vi "ExecuteMenuCommand.vi"(0 "reference in":refnum<class "VINode.lvclass">, 1 "Command":string, 5 "error in (no error)":errorcluster) -> (14 "reference out":refnum<class "VINode.lvclass">, 15 "EditorAction":T3, 16 "FlattenCommandSettings":T1, 19 "error out":errorcluster)   [LabVIEW 2014, in "VINode.lvclass"]
uses:
  <resource>/Framework/Providers/Open_GDS/UML/VINode_class/VINode.lvclass
  <resource>/Framework/Providers/Open_GDS/UML/UMLEditor/UMLEditor EditorActionType.ctl
  <resource>/Framework/Providers/Open_GDS/UML/UMLEditor/UMLEditor FlattenCommandType.ctl
  <resource>/Framework/Providers/Open_GDS/UML/UMLEditor/UMLEditor ExecuteCommandType.ctl
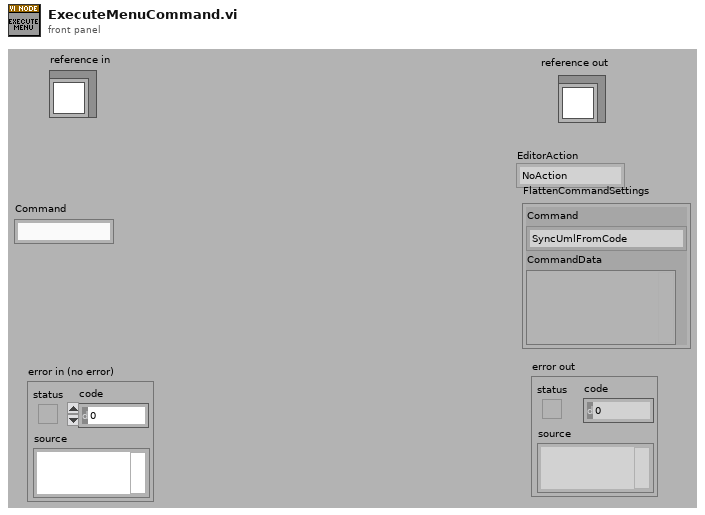
[diagram p1: front panel]
types:
  T1 = typedef "UMLEditor FlattenCommandType.ctl" = cluster{"Command":T2, "CommandData":variant}
  T2 = typedef "UMLEditor ExecuteCommandType.ctl" = enum16{"SyncUmlFromCode", "SyncCodeFromUML", "OpenClass", "OpenFile", "CreateClass", "CreateVI", "OpenClassAttribute", "LocateInProject"}
  T3 = typedef "UMLEditor EditorActionType.ctl" = enum16{"NoAction", "Repaint", "ExecuteCommand"}
  T4 = typedef "VINode.lvclass/ObjectAttributes.ctl" = cluster{"midHeight":dbl, "botHeight":dbl, "Name":refnum<class "MultiLineString.lvclass">, "DEFAULT_COMPARTMENT_HEIGHT":i32, "DEFAULT_WIDTH":i32, "DEFAULT_HEIGHT":i32, "ClassPath":path, "Icon":u8[][], "Description":refnum<class "MultiLineString.lvclass">, "ShowDescription":bool}
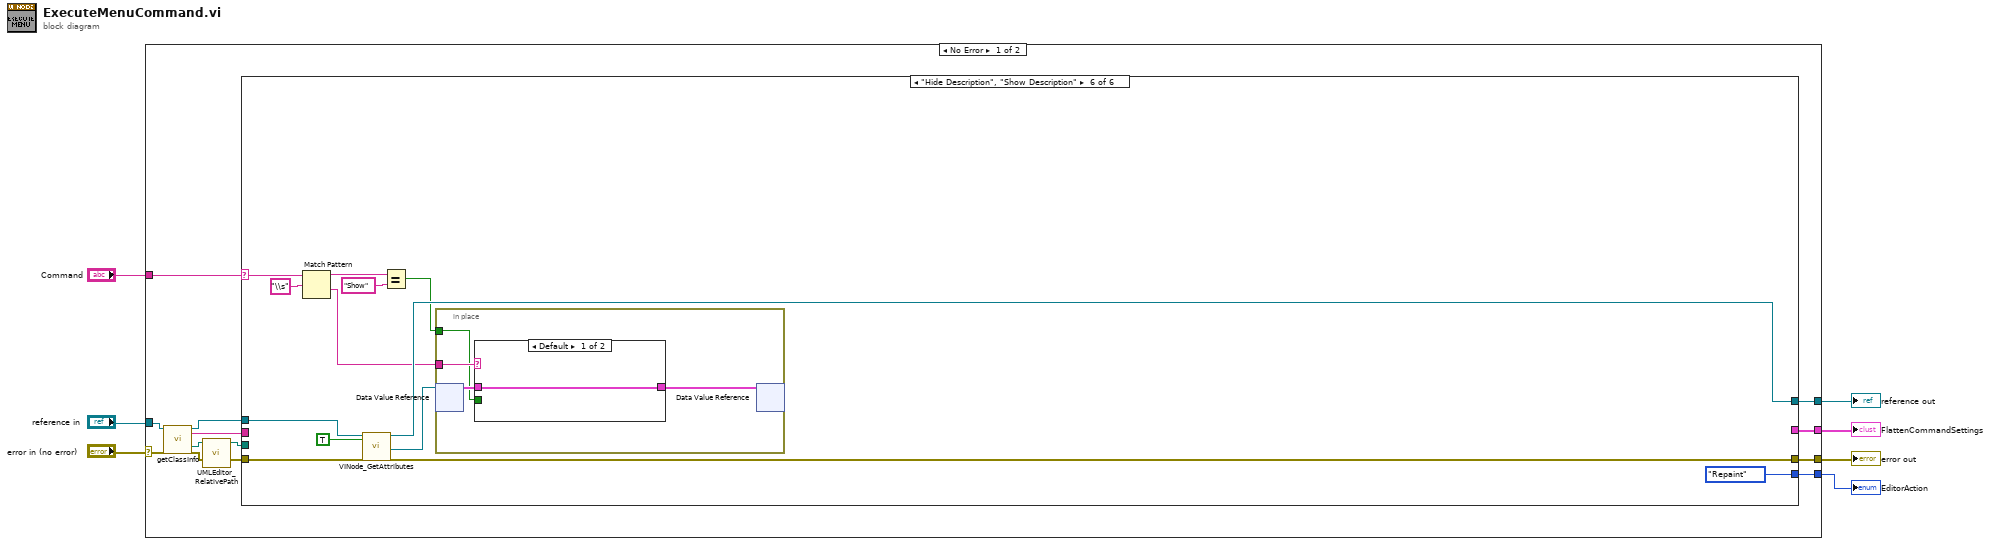
[diagram p0: block diagram]
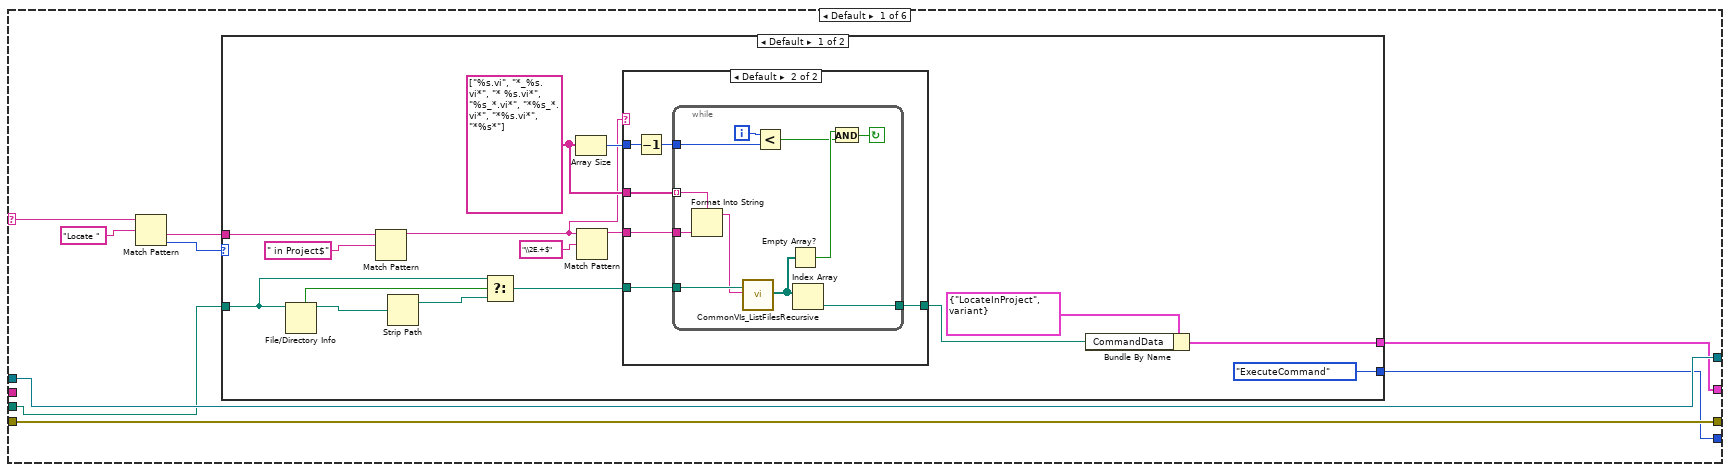
[diagram p2: hidden frame]
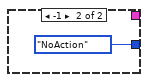
[diagram p4: hidden frame]
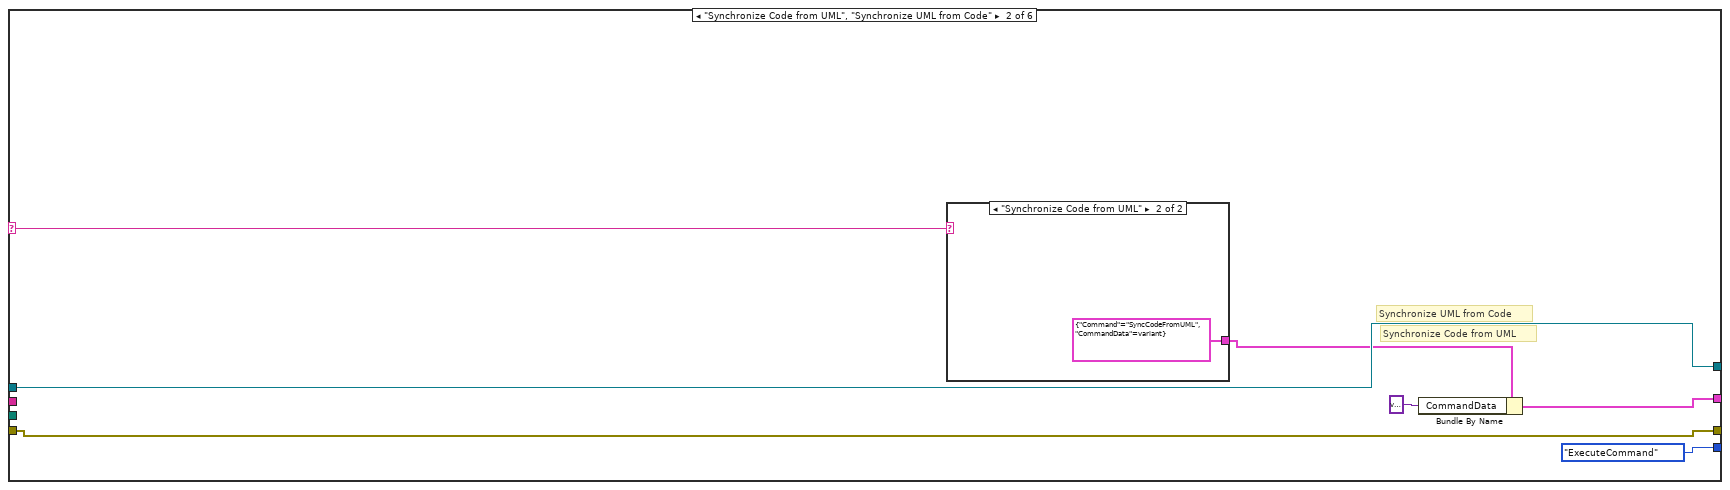
[diagram p5: hidden frame]
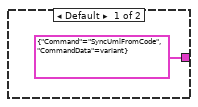
[diagram p6: hidden frame]
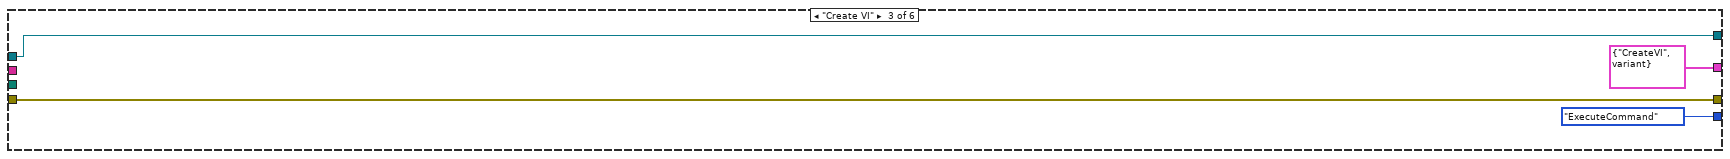
[diagram p7: hidden frame]
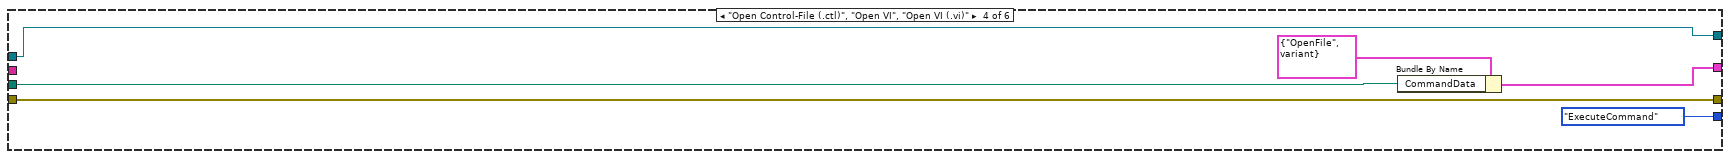
[diagram p8: hidden frame]
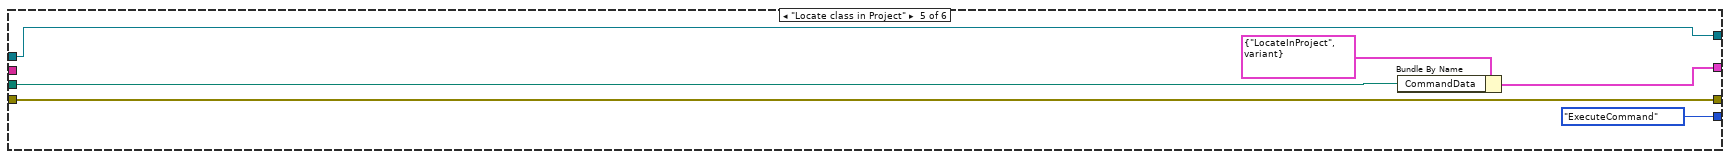
[diagram p9: hidden frame]
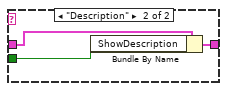
[diagram p10: hidden frame]
diagram:
  n1 = case shown="No Error" "error in (no error)" {
    selector: "error in (no error)" -> [w12 w109]
    tunnel: "reference in" -> [w14 w110]
    tunnel: [w17 w109] -> w5
    tunnel: [w18 w110] -> w4
    tunnel: "Command" -> [w19 _]
    tunnel: [w16 _] -> w2
    tunnel: [w15 _] -> w1
    frame No Error {
      n2 = call-dynamic "getClassInfo.vi"("reference in"=w14, "error in (no error)"=w12) -> ("reference out"=w13:refnum<class "VINode.lvclass">, "className"=w10:string, "ModulePath"=w9:path, "error out"=w11:errorcluster)  [unwired: 12 in, 2 out]
      n3 = call <resource>:"UMLEditor_RelativePath.vi"("Path In"=w9) -> ("ConvertToAbsolutePath(If possible)"=w8:path)  [unwired: 1 in, 17 out]
      n4 = case shown="\"Hide Description\", \"Show Description\"" w19 {
        selector: w19 -> [w25 w63 _ _ _ w95]
        tunnel: w11 -> [w27 w67 w72 w79 w85 w97]
        tunnel: w13 -> [w28 w68 w73 w80 w86 w99]
        tunnel: [w28 w68 w73 w80 w86 w98] -> w18
        tunnel: [w27 w67 w72 w79 w85 w96] -> w17
        tunnel: [w26 UMLEditor_EditorActionType."ExecuteCommand" ("EditorAction") UMLEditor_EditorActionType."ExecuteCommand" ("EditorAction") UMLEditor_EditorActionType."ExecuteCommand" ("EditorAction") UMLEditor_EditorActionType."ExecuteCommand" ("EditorAction") UMLEditor_EditorActionType."Repaint" ("EditorAction")] -> w16
        tunnel: [w21 w65 T1 {"Command"=enum."CreateVI", "CommandData"=variant} ("FlattenCommandSettings") w77 w83 _] -> w15
        tunnel: w8 -> [w20 _ _ w76 w82 _]
        tunnel: w10 -> [_ _ _ _ _ _]
        frame Default {
          n5 = Match Pattern(string=w25, regular expression="Locate ") -> (after substring=w22:string, offset past match=w23:i32)  [unwired: 1 in, 2 out]
          n6 = case shown="Default" w23 {
            tunnel: [UMLEditor_EditorActionType."ExecuteCommand" ("EditorAction") UMLEditor_EditorActionType."NoAction" ("EditorAction")] -> w26
            tunnel: w22 -> [w44 _]
            tunnel: [w40 _] -> w21
            tunnel: w20 -> [w30 _]
            frame Default {
              w35 = string[] ["%s.vi", "*_%s.vi*", "* %s.vi*", "%s_*.vi*", "*%s_*.vi*", "*%s.vi*", "*%s*"]
              n7 = File/Directory Info(path=w30) -> (path out=w33:path, directory=w38:bool)  [unwired: 1 in, 5 out]
              n8 = Match Pattern(string=w44, regular expression=" in Project$") -> (before substring=w31:string)  [unwired: 1 in, 3 out]
              n9 = Strip Path(path=w33) -> (stripped path=w32:path)  [unwired: 1 out]
              n10 = Select(t=w30, s=w38, f=w32) -> (s? t:f=w37:path)
              n11 = Array Size(array=w35) -> (size(s)=w34:i32)
              n12 = Match Pattern(string=w31, regular expression="\\2E.+$") -> (before substring=w36:string)  [unwired: 4 out]
              n13 = case shown="Default" w31 {
                tunnel: [_ w47] -> w29
                tunnel: w37 -> [_ w50]
                tunnel: w35 -> [_ w49]
                tunnel: w36 -> [_ w48]
                tunnel: w34 -> [_ w46]
                frame "" {
                }
                frame Default {
                  n14 = Decrement(x=w46) -> (x-1=w45:i32)
                  n15 = while {
                    tunnel: w50 -> [w61]
                    tunnel: w49 -> [w60] mode=indexing
                    tunnel: w48 -> [w59]
                    tunnel: [w58] -> w47
                    tunnel: w45 -> [w54]
                    i -> [w55]
                    stop <- w51 continue-if-true
                    n16 = Format Into String(format string=w60, w59) -> (resulting string=w56:string)  [unwired: 2 in, 1 out]
                    n17 = call <resource>:"CommonVIs_ListFilesRecursive.vi"("directory path"=w61, "FileSearchPattern"=w56) -> ("Files"=w57:path[])  [unwired: 4 in, 13 out]
                    n18 = Less?(x=w55, y=w54) -> (x < y?=w52:bool)
                    n19 = Empty Array?(array=w57) -> (empty?=w53:bool)
                    n20 = Index Array(array=w57) -> (element=w58:path)  [unwired: 1 in]
                    n21 = And(x=w53, y=w52) -> (x .and. y?=w51:bool)
                  }
                }
              }
              n22 = Bundle By Name(cluster=T1 {"Command"=enum."LocateInProject", "CommandData"=variant} ("FlattenCommandSettings"), "CommandData"=w29) -> (w40:T1)
            }
            frame -1 {
            }
          }
        }
        frame "Synchronize Code from UML", "Synchronize UML from Code" {
          # "Synchronize Code from UML"
          # "Synchronize UML from Code"
          n23 = case shown="\"Synchronize Code from UML\"" w63 {
            tunnel: [T1 {"Command"=enum."SyncUmlFromCode", "CommandData"=variant} ("FlattenCommandSettings") T1 {"Command"=enum."SyncCodeFromUML", "CommandData"=variant} ("FlattenCommandSettings")] -> w66
            frame Default {
            }
            frame "Synchronize Code from UML" {
            }
          }
          n24 = Bundle By Name(cluster=w66, "CommandData"=variant) -> (w65:T1)
        }
        frame "Create VI" {
        }
        frame "Open Control-File (.ctl)", "Open VI", "Open VI (.vi)" {
          n25 = Bundle By Name(cluster=T1 {"Command"=enum."OpenFile", "CommandData"=variant} ("FlattenCommandSettings"), "CommandData"=w76) -> (w77:T1)
        }
        frame "Locate class in Project" {
          n26 = Bundle By Name(cluster=T1 {"Command"=enum."LocateInProject", "CommandData"=variant} ("FlattenCommandSettings"), "CommandData"=w82) -> (w83:T1)
        }
        frame "Hide Description", "Show Description" {
          n27 = Match Pattern(string=w95, regular expression="\\s") -> (before substring=w91:string, after substring=w89:string)  [unwired: 3 out]
          n28 = call <resource>:"VINode_GetAttributes.vi"("reference in"=w99, "OnlyGetDvrReference(False)"=TRUE, "error in (no error)"=w97) -> ("reference out"=w98:refnum<class "VINode.lvclass">, "DataRef"=w90:refnum<data-value>, "error out"=w96:errorcluster)  [unwired: 13 in, 1 out]
          n29 = Equal?(x=w91, y="Show") -> (x = y?=w88:bool)
          n30 = in-place {
            in-place-border: w89 -> [w104]
            in-place-border: w88 -> [w102]
            n31 = in-place-dvr #1(w90) -> (w103:T4)  [unwired: 1 out]
            n32 = case shown="Default" w104 {
              tunnel: w103 -> [w105 w108]
              tunnel: [w105 w107] -> w101
              tunnel: w102 -> [_ w106]
              frame Default {
              }
              frame "Description" {
                n33 = Bundle By Name(cluster=w108, "ShowDescription"=w106) -> (w107:T4)
              }
            }
            n34 = in-place-dvr #1(w101) -> ()  [unwired: 2 out]
          }
        }
      }
    }
    frame Error {
    }
  }
  "reference out" <- w4
  "error out" <- w5
  "FlattenCommandSettings" <- w1
  "EditorAction" <- w2
